vi "Dashboard Main.vi"() -> ()   [LabVIEW 2019]
uses:
  <vilib>/Utility/miscctls.llb/LVRowAndColumnTypeDef.ctl
  <vilib>/event_ctls.llb/eventvkey.ctl
  <vilib>/Rock Robotics/Network Tables/NT Read Numeric Array.vi
  <vilib>/Rock Robotics/WPI/Dashboard/WPI_DashboardLogging Global.vi
panel:
  in  "On/Off  2":bool caption="Solenoid"
  in  "On/Off  2":bool caption="Solenoid"
  in  "On/Off  2":bool caption="Solenoid"
  in  "On/Off  2":bool caption="Solenoid"
  in  "Camera Settings Right":T1={"Frame Rate"=30, "Compression"=30, "Size"=1, "DB Camera Config"=FALSE} {"Frame Rate" scale=1.0..30.0; "Compression" scale=100.0..-1.0; "Size" items=["640x480", "320x240", "160x120"]}
  in  "Camera Name Right":string(combo)="No Camera Selection"
  out "Camera Perf":string
  in  "Camera Settings":T1={"Frame Rate"=30, "Compression"=30, "Size"=1, "DB Camera Config"=FALSE} {"Frame Rate" scale=1.0..30.0; "Compression" scale=100.0..-1.0; "Size" items=["640x480", "320x240", "160x120"]}
  in  "TCP":refnum<k5>
  in  "Rec Mode":enum32{"Stop", "Record", "Playback"}(radio)
  out "Robot IP":string
  out "Image Message":string="Timeout in Camera Communications"
  in  "Dashboard Tab":T2(tab)
  in  "Select Auto":string(combo)="Select Autonomous ..."
  out "NT Connection":bool
  out "MotorChart R":cluster{"Numeric":dbl, "Numeric":dbl}(graph)
  out "MotorChart L":cluster{"Numeric":dbl, "Numeric":dbl}(graph)
  out "MotorSliders R":cluster{"MotorSlide1":dbl, "MotorSlide2":dbl} {"MotorSlide2" scale=-1.0..1.0 scale format="%#_2e"; "MotorSlide1" scale=-1.0..1.0 scale format="%#_2e"}
  out "MotorSliders L":cluster{"MotorSlide1":dbl, "MotorSlide2":dbl} {"MotorSlide2" scale=-1.0..1.0 scale format="%#_2e"; "MotorSlide1" scale=-1.0..1.0 scale format="%#_2e"}
  out "Gyro":dbl(knob) scale=0.0..360.0
  out "JS1 Z":dbl(slide) scale=-1.0..1.0 scale format="%#_2e"
  out "JS1 Graph":cluster{"X":dbl, "Y":dbl}[](graph)
  out "JS1 Buttons":T3
  out "JS2 Z":dbl(slide) scale=-1.0..1.0 scale format="%#_2e"
  out "JS2 Graph":cluster{"X":dbl, "Y":dbl}[](graph)
  out "JS2 Buttons":T3
  out "Mode":T4(ring)=enum."Auto Disabled"
  out "Right Camera Perf":cluster{"Bandwidth (Mbps)":dbl, "FPS":dbl}
  out "Camera Image Right":T5(plugin-control)
  in  "DB/String 9":string
  in  "DB/String 8":string
  in  "DB/String 7":string
  in  "DB/String 6":string
  in  "DB/String 5":string
  in  "DB/String 4":string
  in  "DB/String 3":string
  in  "DB/String 2":string
  in  "DB/String 1":string
  in  "DB/String 0":string
  in  "DB/Slider 0":dbl(slide) scale=0.0..5.0
  in  "DB/Slider 1":dbl(slide) scale=0.0..5.0
  in  "DB/Slider 2":dbl(slide) scale=0.0..5.0
  in  "DB/Slider 3":dbl(slide) scale=0.0..5.0
  out "DB/LED 3":bool
  out "DB/LED 2":bool
  out "DB/LED 1":bool
  out "DB/LED 0":bool
  in  "DB/Button 3":bool
  in  "DB/Button 2":bool
  in  "DB/Button 1":bool
  in  "DB/Button 0":bool caption="New Name"
  in  "Auto Elevator":bool
  out "Current Color":string
  out "Current Trim":dbl
  in  "Trim Start":dbl
  out "Shooter Trim":string
  out "In Camera":bool
  out "No Current Draw":string
  out "Over 250 Amps":bool
  out "Aligned":bool
  out "Wheel at Speed":bool
  out "Ready to Fire":bool
  in  "Auton Delay":dbl
  in  "Autonomous":string(combo)
  out "Elevator Sensor":dbl
  in  "p input":dbl
  out "Left Drive Encoder":string
  out "Shooter Encoder":string
  out "Gyro":string
  out "Limelight-Distance":string
  out "Limelight-TS":string
  out "Limelight-TY":string
  out "Limelight-TX":string
  out "Control Panel Color Sensor":string
  out "Control Panel Encoder":string
  out "Right Drive Encoder":string
  out "Conveyor Motor":string
  out "Right Climber":string
  out "Left Climber":string
  out "Buddy Climb Motor":string
  out "Intake Motor":string
  out "Shooter Motor 2":string
  out "Shooter Motor 1":string
  out "Control Panel":string
  out "Right Drive Motor 2":string
  out "Right Drive Motor 1":string
  out "Left Drive Motor 2":string
  out "Left Drive Motor 1":string
  in  "Test Slider":dbl(slide) scale=0.0..100.0 scale format="%#_3g"
  in  "On/Off":bool caption="Solenoid"
  in  "Test Name":u16(ring) items=["Select the test to run..."]
  in  "Test Tree":string(tree)
  in  "Motor":cluster{"Value":dbl, "Enable":bool} {"Value" scale=-1.0..1.0 scale format="%#_3g"}
  out "Progress":T6 {"Test Progress" scale=0.0..100.0}
  in  "Rev/Fwd":cluster{"Forward":bool, "Reverse":bool}
  in  "Test Ring":u16(ring) items=["Monochrome", "Color"]
  out "Cmd Status":string
  in  "Execute Command":bool
  in  "Command Params":string[][](table)
  in  "Command Selection":i32(listbox)
  in  "CheckList":i32(listbox)
  out "Tree":string(tree)
  out "Camera Image":T5(plugin-control)
  in  "Camera Name":string(combo)="No Camera Selection"
  # "HW"
  # "HW"
  # "Joysticks"
  # "Drive Motors"
  # "Front"
  # "Right"
  # "Left"
  # "Back"
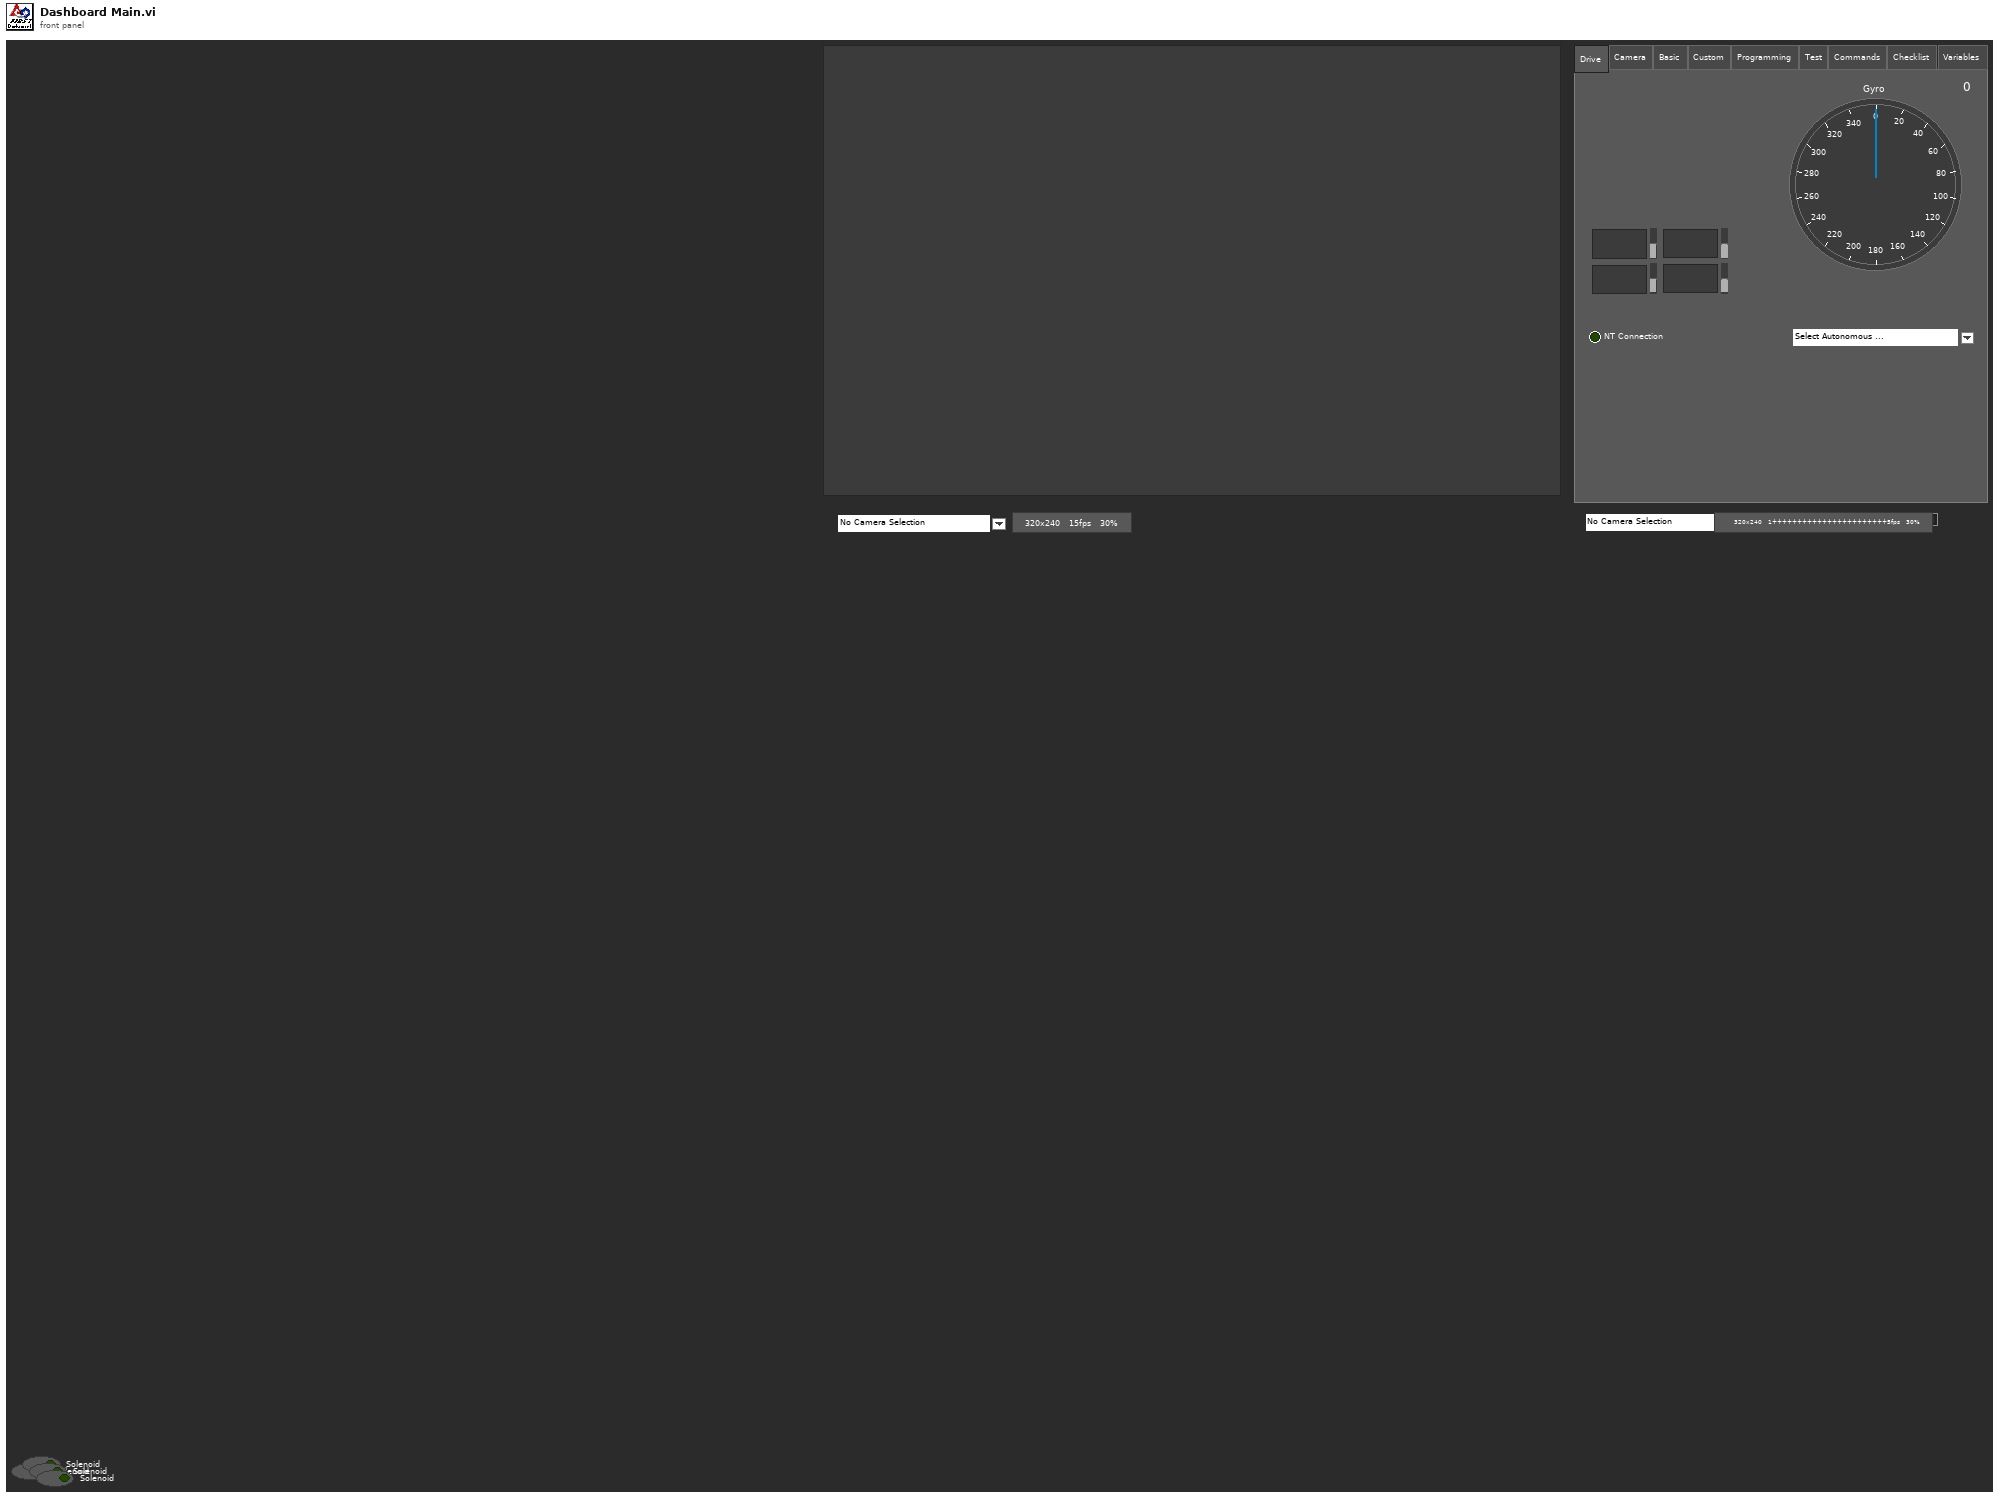
[diagram p1: front panel]
types:
  T1 = cluster{"Frame Rate":i32, "Compression":i32, "Size":u16, "DB Camera Config":bool}
  T2 = enum32{"Drive", "Camera", "Basic", "Custom", "Programming", "Test", "Commands", "Checklist", "Variables"}
  T3 = cluster{bool, bool, bool, bool, bool, bool, bool, bool, bool, bool, bool, bool}
  T4 = enum8{"Tele-Op Disabled", "Tele-Op Enabled", "Auto Disabled", "Auto Enabled", "Test Disabled", "Test Enabled", "Disconnected", "No Code", "E-Stop"}
  T5 = typedef "IMAQ Image.ctl" = refnum<image>
  T6 = cluster{"Test Progress":u8, "Test Progress Text":string}
  T7 = enum32{"Drive", "Camera", "Basic", "Programming", "Custom", "Test", "Commands", "Checklist", "Variables"}
  T8 = cluster{"Save Path":path, "Interval (s)":dbl, "Keep":i32}
  T9 = typedef "Image Type" = u32
  T10 = cluster{"IDs":cluster{"RPC field ID":u16, "Unique ID":u16}, "String":string}
  T11 = cluster{"Error Strings":string, "Disable Counts":cluster{u16, u16}, "Rail Faults":cluster{u16, u16, u16}, "Robot IP":string, "DB Mode":u8, "Event Info":cluster{"Name":string, "Type":u8, "Number":u16, "Replay":u8}}
  T12 = cluster{"Storage":cluster{"Disk Free":u64, "RAM Block":u32, "RAM free":u32}, "CPU Utilization":cluster{"CPU % ISR":sgl, "CPU % Time Crit":sgl, "CPU % Timed Str":sgl, "CPU % High":sgl, "CPU % Above":sgl, "CPU % Normal":sgl, "CPU % Low":sgl}, "CAN":cluster{"% Bus Utilization":sgl, "Bus Off Cnt":u32, "TX_FIFO Full Cnt":u32, "Receive Error Cnt":u8, "Transmit Error Cnt":u8}, "HID":cluster{"HID Outputs":u32, "Rumble Low":u16, "Rumble High":u16}[]}
  T13 = cluster{"Status bits":cluster{"Test Mode":bool, "Autonomous":bool, "Enabled":bool, "Code Start":bool, "Brownout":bool, "Reserved 2":bool, "Reserved 3":bool, "E-Stop":bool}, "Code Trace":cluster{"Disabled":bool, "TeleOp":bool, "Auto":bool, "Test":bool}, "Controller Type":enum16{"unknown", "cRIO", "roboRio"}, "Code?":enum16{"unknown", "noCode", "code"}, "Battery V":dbl}
  T14 = cluster{"Control Bits":cluster{"TestMode":bool, "Autonomous":bool, "Enabled":bool, "FMS Present":bool, bool, bool, bool, "E-Stop":bool}, "Team Station ":u8, "Countdown":sgl, "Joystick Values":cluster{"Axes":dbl[], "Buttons":bool[], "POVs":i16[]}[]}
  T15 = cluster{"Axes":dbl[], "Buttons":bool[], "POVs":i16[]}[]
  T16 = cluster{"Axes":dbl[], "Buttons":bool[], "POVs":i16[]}
  T17 = cluster{"Buttons[0]":bool, "Buttons[1]":bool, "Buttons[2]":bool, "Buttons[3]":bool, "Buttons[4]":bool, "Buttons[5]":bool, "Buttons[6]":bool, "Buttons[7]":bool, "Buttons[8]":bool, "Buttons[9]":bool, "Buttons[10]":bool, "Buttons[11]":bool}
  T18 = cluster{"Camera Image":refnum<vi>, "Dashboard Tab":refnum<vi>, "Background":refnum<vi>, "Rec Mode":refnum<vi>, "Test Slider":refnum<vi>, "On/Off ":refnum<vi>, "Test Ring":refnum<vi>, "Rev/Fwd":refnum<vi>, "Test Name":refnum<vi>, "Motor":refnum<vi>, "Progress":refnum<vi>, "CheckList":refnum<vi>, "Tree":refnum<vi>, "Test Tree":refnum<vi>, "Command Params":refnum<vi>, "Command Selection":refnum<vi>, "Execute Command":refnum<vi>, "Cmd Status":refnum<vi>, "Camera Settings":refnum<vi>, "Camera Name":refnum<vi>, "Camera Perf":refnum<vi>, "Camera Settings Right":refnum<vi>, "Camera Name Right":refnum<vi>, "Camera Image Right":refnum<vi>}
  T19 = cluster{"Global Rectangle":i32[], "Contours":cluster{"Contour Type":u32, "ROI Type":u32, "Points":i32[]}[]}
  T20 = cluster{"Camera Name":string, string, "Saved DB Images Info":cluster{"Save Path":path, "Interval (s)":dbl, "Keep":i32}}
  T21 = cluster{"Camera Name Right":string, string, "Saved DB Images Info":cluster{"Save Path":path, "Interval (s)":dbl, "Keep":i32}}
  T22 = cluster{"Operation":enum16{"Update", "Clear"}, "Color Box":u32}[]
  T23 = typedef "eventvkey.ctl" = enum16{"ASCII", "Enter", "Return", "Shift", "Ctrl", "Alt", "Cmd", "Opt", "Caps", "NumLock", "Clear", "Break", "Up", "Down", "Left", "Right", "Insert", "Delete", "Home", "End", "PageUp", "PageDown", "Escape", "Help", "Pause", "ScrollLock", "F1", "F2", "F3", "F4", "F5", "F6", "F7", "F8", "F9", "F10", "F11", "F12", "F13", "F14", "F15", "F16", "F17", "F18", "F19", "F20", "F21", "F22", "F23", "F24", "Play", "VolumeUp", "VolumeDown", "Mute", "Two Byte Char"}
  T24 = cluster{"Image Size":bool, "Image Type":bool, "Pixel Value":bool, "ROI Information":bool, "Zoom Factor":bool}
  T25 = cluster{"Operation":enum16{"Update", "Clear"}, "Color Box":u32}
  T26 = typedef "LVRowAndColumnTypeDef.ctl" = cluster{"Row":i32, "Column":i32}
  T27 = cluster{"Shift":bool, "Ctrl":bool, "Alt":bool, "Cmd":bool, "Opt":bool}
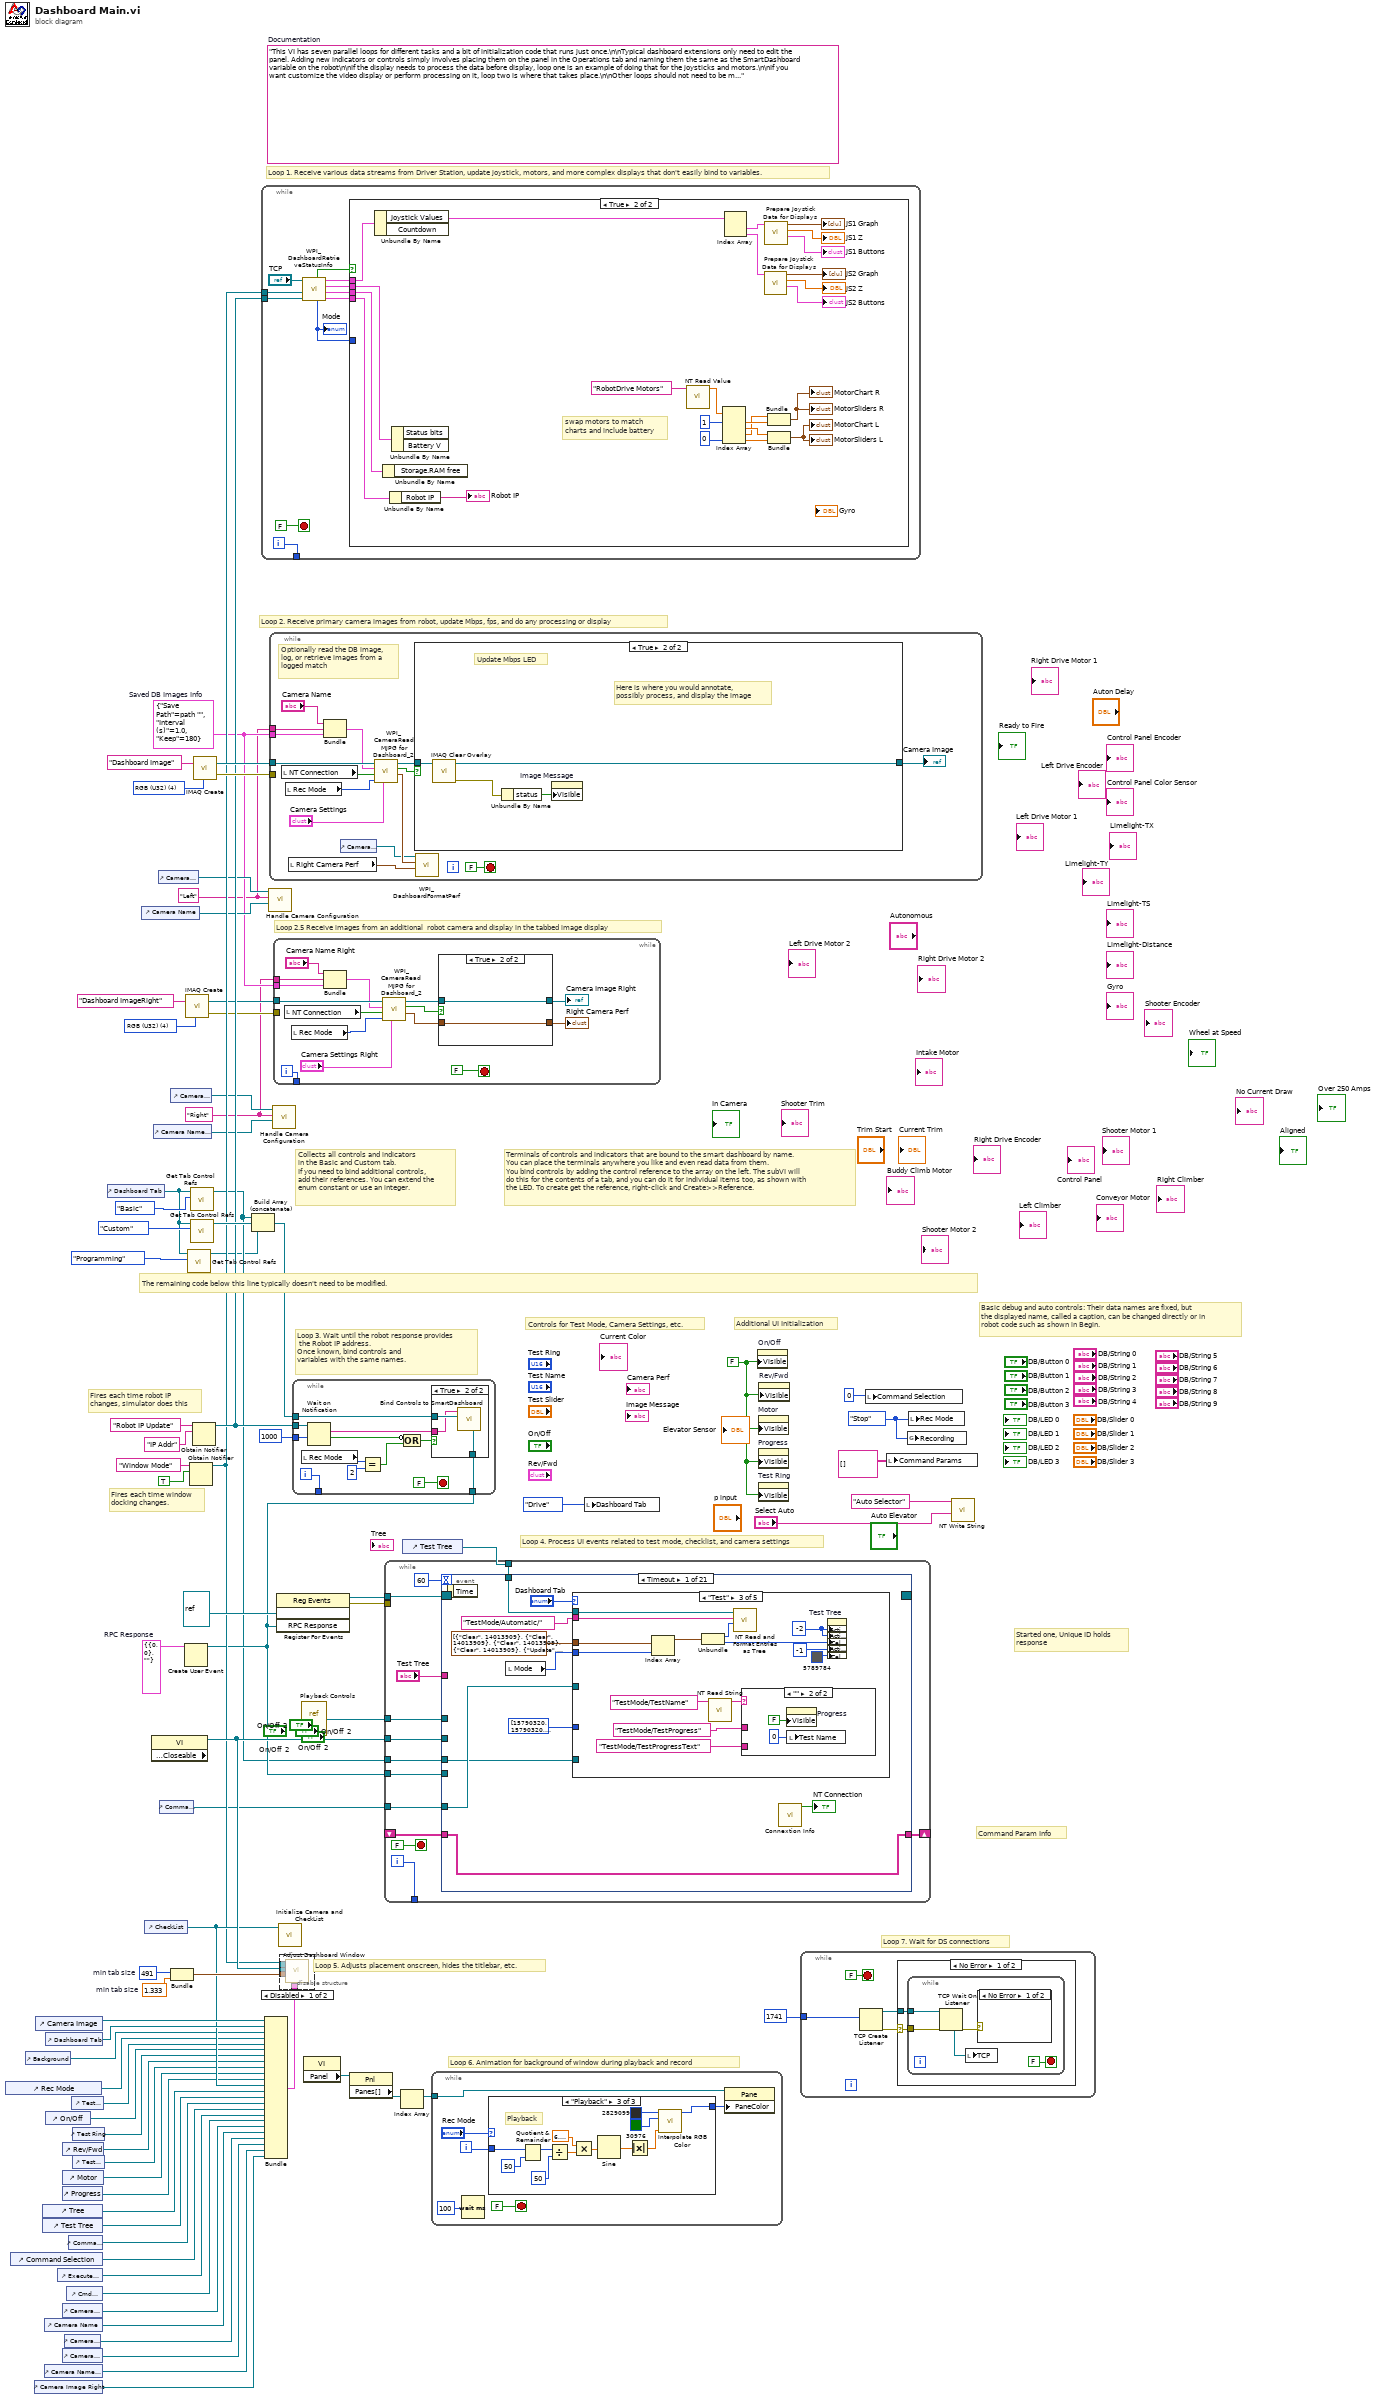
[diagram p0: block diagram]
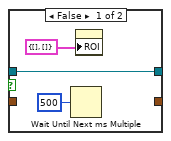
[diagram p3: hidden frame]
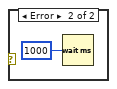
[diagram p4: hidden frame]
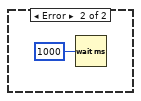
[diagram p5: hidden frame]
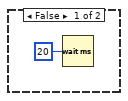
[diagram p6: hidden frame]
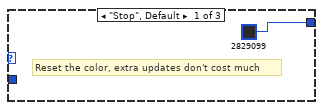
[diagram p7: hidden frame]
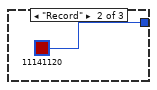
[diagram p8: hidden frame]
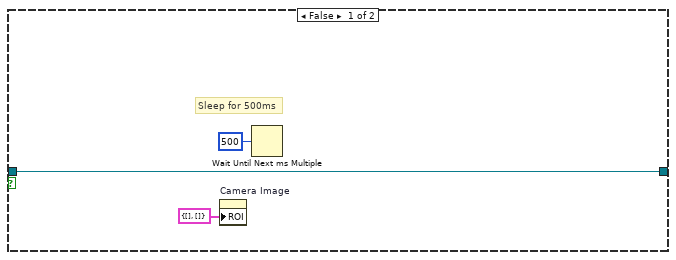
[diagram p10: hidden frame]
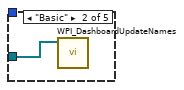
[diagram p12: hidden frame]
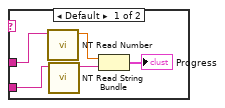
[diagram p13: hidden frame]
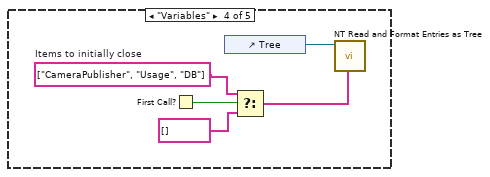
[diagram p14: hidden frame]
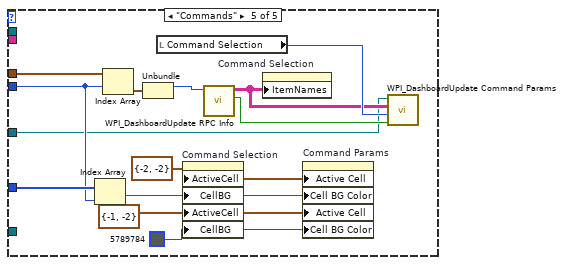
[diagram p15: hidden frame]
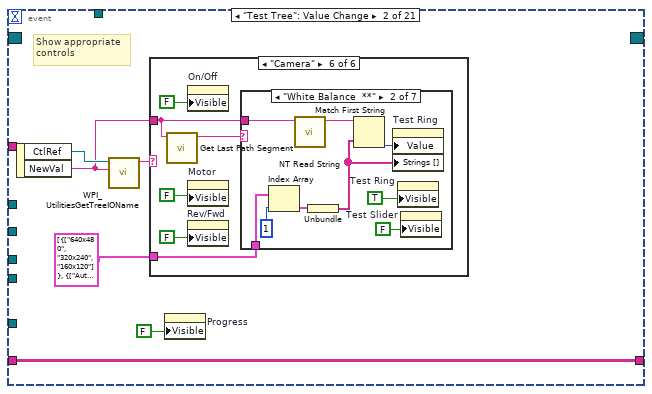
[diagram p16: hidden frame]
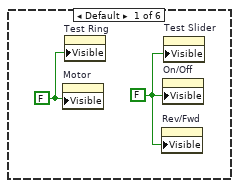
[diagram p17: hidden frame]
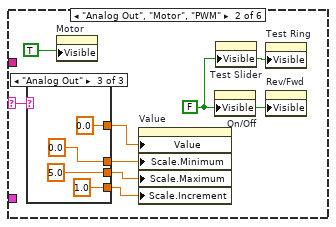
[diagram p18: hidden frame]
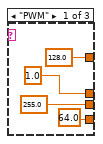
[diagram p19: hidden frame]
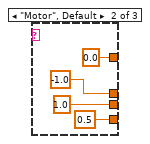
[diagram p20: hidden frame]
diagram:
  w7 = T8 {"Save Path"=path "", "Interval (s)"=1.0, "Keep"=180}  # Saved DB Images Info
  w6 = "Right"
  w5 = "Left"
  w17 = T9 4 items=["Grayscale (U8)", "Grayscale (I16)", "Grayscale (SGL)", "Complex (CSG)", "RGB (U32)", "HSL (U32)", "RGB (U64)"] ("Image Type")
  w33 = T10 {"IDs"={"RPC field ID"=0, "Unique ID"=0}, "String"=""}  # RPC Response
  w55 = 491  # min tab size
  w54 = 1.333  # min tab size
  w61 = enum32{"Stop", "Record", "Playback"}."Stop" ("Rec Mode")
  w40 = FALSE ("Visible")
  (unwired) "This VI has seven parallel loops for different tasks and a bit of initialization code that runs just once.\n\nTypical dashboard extensions only need to edit the panel. Adding new indicators or controls simply involves placing them on the panel in the Operations tab and naming them the same as the SmartDashboard variable on the robot\n\nIf the display needs to process the data before display, loop one is an example of doing that for the joysticks and motors.\n\nIf you want customize the video display or perform processing on it, loop two is where that takes place.\n\nOther loops should not need to be modified. They are pretty standard, and document the task they perform."  # Documentation
  w78 = T9 4 items=["Grayscale (U8)", "Grayscale (I16)", "Grayscale (SGL)", "Complex (CSG)", "RGB (U32)", "HSL (U32)", "RGB (U64)"] ("Image Type")
  # "Loop 2.5 Receive images from an additional  robot camera and display in the tabbed image display"
  # "Command Param Info"
  # "Started one, Unique ID holds\nresponse"
  # "Loop 7. Wait for DS connections"
  # "Basic debug and auto controls: Their data names are fixed, but\nthe displayed name, called a caption, can be changed directly or in\nrobot code such as shown in Begin."
  # "Controls for Test Mode, Camera Settings, etc."
  # "Additional UI Initialization"
  # "Loop 6. Animation for background of window during playback and record"
  # "Fires each time robot IP\nchanges, simulator does this"
  # "Fires each time window\ndocking changes."
  # "Collects all controls and indicators\nin the Basic and Custom tab.\nIf you need to bind additional controls,\nadd their references. You can extend the\nenum constant or use an integer."
  # "The remaining code below this line typically doesn't need to be modified."
  # "Loop 4. Process UI events related to test mode, checklist, and camera settings"
  # "Terminals of controls and indicators that are bound to the smart dashboard by name.\nYou can place the terminals anywhere you like and even read data from them.\nYou bind controls by adding the control reference to the array on the left. The subVI will\ndo this for the contents of a tab, and you can do it for individual items too, as shown with\nthe LED. To create get the reference, right-click and Create>>Reference."
  # "Loop 3. Wait until the robot response provides\n the Robot IP address.\nOnce known, bind controls and\nvariables with the same names."
  # "Loop 5. Adjusts placement onscreen, hides the titlebar, etc."
  # "Loop 1. Receive various data streams from Driver Station, update joystick, motors, and more complex displays that don't easily bind to variables."
  # "Loop 2. Receive primary camera images from robot, update Mbps, fps, and do any processing or display"
  n1 = control-ref of="Rec Mode"() -> (w46:refnum<vi>)
  n2 = control-ref of="Command Selection"() -> (w32:refnum<vi>)
  n3 = control-ref of="Background"() -> (w4:refnum<vi>)
  n4 = control-ref of="Camera Image Right"() -> (w10:refnum<vi>)
  n5 = control-ref of="Camera Image"() -> (w57:refnum<vi>)
  n6 = control-ref of="Tree"() -> (w50:refnum<vi>)
  n7 = control-ref of="Test Tree"() -> (w49:refnum<vi>)
  n8 = control-ref of="Camera Name"() -> (w23:refnum<vi>)
  n9 = control-ref of="Camera Name Right"() -> (w11:refnum<vi>)
  n10 = control-ref of="On/Off"() -> (w44:refnum<vi>)
  n11 = control-ref of="Dashboard Tab"() -> (w56:refnum<vi>)
  n12 = control-ref of="Execute Command"() -> (w34:refnum<vi>)
  n13 = control-ref of="Progress"() -> (w41:refnum<vi>)
  n14 = control-ref of="Camera Settings"() -> (w24:refnum<vi>)
  n15 = control-ref of="Camera Settings Right"() -> (w12:refnum<vi>)
  n16 = control-ref of="Rev/Fwd"() -> (w42:refnum<vi>)
  n17 = control-ref of="Motor"() -> (w47:refnum<vi>)
  n18 = control-ref of="Camera Perf"() -> (w22:refnum<vi>)
  n19 = control-ref of="Cmd Status"() -> (w28:refnum<vi>)
  n20 = control-ref of="Command Params"() -> (w35:refnum<vi>)
  n21 = control-ref of="Test Slider"() -> (w45:refnum<vi>)
  n22 = control-ref of="Test Ring"() -> (w43:refnum<vi>)
  n23 = control-ref of="Test Name"() -> (w48:refnum<vi>)
  n24 = control-ref of="Dashboard Tab"() -> (w2:refnum<vi>)
  n25 = control-ref of="Camera Name"() -> (w25:refnum<vi>)
  n26 = control-ref of="CheckList"() -> (w51:refnum<vi>)
  n27 = property class="VI" props=["Front Panel.Closeable"]() -> (reference out=w60:refnum<vi>)  [unwired: 2 in, 2 out]
  n28 = control-ref of="Camera Name Right"() -> (w13:refnum<vi>)
  n29 = control-ref of="Camera Settings"() -> (w26:refnum<vi>)
  n30 = control-ref of="Command Params"() -> (w27:refnum<vi>)
  n31 = control-ref of="Camera Settings Right"() -> (w14:refnum<vi>)
  n32 = Bundle("min tab size"=w55, "min tab size"=w54) -> (w53:cluster{"min tab size":i32, "min tab size":dbl})  [unwired: 1 in]
  n33 = Create User Event(user event datatype=w33) -> (user event=w29:refnum<user-event>)  [unwired: 1 in, 1 out]
  n34 = call "IMAQ Create"("Image Name"="Dashboard ImageRight", "Image Type"=w17) -> ("New Image"=w16:T5, "error out"=w15:errorcluster)  [unwired: 2 in, 1 out]
  n35 = call <vilib>:"Get Tab Control Refs.vi"("Page Index"=T7."Programming" ("Dashboard Tab"), "TabControl in"=w2) -> ("ControlsOnPage"=w1:refnum<vi>[])  [unwired: 9 in]
  n36 = Obtain Notifier(name (unnamed)="Window Mode", notification data type=TRUE) -> (notifier out=w38:refnum<notifier>)  [unwired: 2 in, 2 out]
  n37 = call <vilib>:"Get Tab Control Refs.vi"("Page Index"=T7."Basic" ("Dashboard Tab"), "TabControl in"=w2) -> ("ControlsOnPage"=w21:refnum<vi>[])  [unwired: 9 in]
  n38 = call <vilib>:"Get Tab Control Refs.vi"("Page Index"=T7."Custom" ("Dashboard Tab"), "TabControl in"=w2) -> ("ControlsOnPage"=w59:refnum<vi>[])  [unwired: 9 in]
  n39 = Obtain Notifier(name (unnamed)="Robot IP Update", notification data type="IP Addr" ("name (unnamed)")) -> (notifier out=w39:refnum<notifier>)  [unwired: 2 in, 2 out]
  n40 = call "IMAQ Create"("Image Name"="Dashboard Image", "Image Type"=w78) -> ("New Image"=w76:T5, "error out"=w75:errorcluster)  [unwired: 2 in, 1 out]
  n41 = Build Array (concatenate)(w21, w59, w1) -> (w58:refnum<vi>[])
  n42 = while {
    tunnel: [w88] -> _
    tunnel: w39 -> [w82]
    tunnel: w38 -> [w79]
    i -> [w88]
    stop <- FALSE stop-if-true
    n43 = call <vilib>:"WPI_DashboardRetrieveStatusInfo.vi"("Binding Refnum"=w82, "Window Mode Notifier"=w79, "TCP Cnx"="TCP") -> ("Power and Errors"=w83:T11, "Robot Metrics"=w86:T12, "Status Info"=w87:T13, "Control Info"=w84:T14, "Robot Mode"=w81:T4, "Process?"=w85:bool)  [unwired: 3 in]
    "Mode" <- w81
    n44 = case shown="True" w85 {
      tunnel: w87 -> [_ w114]
      tunnel: w86 -> [_ w113]
      tunnel: w84 -> [_ w112]
      tunnel: w83 -> [_ w111]
      tunnel: w81 -> [_ _]
      frame False {
        n45 = Wait (ms)(milliseconds to wait=u32 20) -> ()  [unwired: 1 out]
      }
      frame True {
        # "swap motors to match\ncharts and include battery"
        n46 = Unbundle By Name(w112) -> ("Joystick Values"=w102:T15)  [unwired: 1 out]
        n47 = Unbundle By Name(w113) -> ()  [unwired: 1 out]
        n48 = Unbundle By Name(w111) -> ("Robot IP"=→"Robot IP":string)
        n49 = Unbundle By Name(w114) -> ()  [unwired: 2 out]
        n50 = call-poly <vilib>:"NT Read Value.vi"("Name"="RobotDrive Motors") -> ("Numeric Array"=w92:dbl[])  [unwired: 9 in, 1 out]
        n51 = Index Array(array=w92, index #1=1, index #4=0) -> (element #1=w106:dbl, element #2=w107:dbl, element #3=w105:dbl, element #4=w110:dbl)  [unwired: 2 in]
        n52 = Index Array(array=w102) -> (element #1=w101:T16, element #2=w97:T16)  [unwired: 2 in]
        n53 = call "Prepare Joystick Data for Displays.vi"("Joystick Values"=w97) -> ("Buttons"=→"JS2 Buttons":T17, "Z Axis"=→"JS2 Z":dbl, "Cartesian Data"=→"JS2 Graph":cluster{"X axis":dbl, "X axis":dbl}[])  [unwired: 8 in]
        n54 = call "Prepare Joystick Data for Displays.vi"("Joystick Values"=w101) -> ("Buttons"=→"JS1 Buttons":T17, "Z Axis"=→"JS1 Z":dbl, "Cartesian Data"=→"JS1 Graph":cluster{"X axis":dbl, "X axis":dbl}[])  [unwired: 8 in]
        n55 = Bundle("Numeric"=w105, "Numeric"=w106) -> (→"MotorChart R" →"MotorSliders R":cluster{"Numeric":dbl, "Numeric":dbl})  [unwired: 1 in]
        n56 = Bundle("Numeric"=w107, "Numeric"=w110) -> (→"MotorChart L" →"MotorSliders L":cluster{"Numeric":dbl, "Numeric":dbl})  [unwired: 1 in]
      }
    }
  }
  n57 = Bundle("Camera Image"=w57, "Dashboard Tab"=w56, "Background"=w4, "Rec Mode"=w46, "Test Slider"=w45, "On/Off"=w44, "Test Ring"=w43, "Rev/Fwd"=w42, "Test Name"=w48, "Motor"=w47, "Progress"=w41, "CheckList"=w51, "Tree"=w50, "Test Tree"=w49, "Command Params"=w35, "Command Selection"=w32, "Execute Command"=w34, "Cmd Status"=w28, "Camera Settings"=w24, "Camera Name"=w23, "Camera Perf"=w22, "Camera Settings Right"=w12, "Camera Name Right"=w11, "Camera Image Right"=w10) -> (w52:T18)  [unwired: 1 in]
  n58 = call "Handle Camera Configuration.vi"("CameraNameRef"=w25, "Display Name"=w5, "ClusterRef"=w26) -> ()  [unwired: 9 in]
  n59 = while {
    tunnel: w76 -> [w128]
    tunnel: w75 -> [_]
    tunnel: w7 -> [w121]
    tunnel: w5 -> [w118]
    stop <- FALSE stop-if-true
    # "Optionally read the DB image,\nlog, or retrieve images from a\nlogged match"
    n60 = local read "NT Connection"() -> (w122:bool)
    n61 = local read "Rec Mode"() -> (w125:enum32{"Stop", "Record", "Playback"})
    n62 = local read "Right Camera Perf"() -> (w116:cluster{"Bandwidth (Mbps)":dbl, "FPS":dbl})
    n63 = Bundle("Camera Name"="Camera Name", w118, "Saved DB Images Info"=w121) -> (w120:T20)  [unwired: 1 in]
    n64 = control-ref of="Camera Perf"() -> (w115:refnum<vi>)
    n65 = call <vilib>:"WPI_CameraRead MJPG for Dashboard_2.vi"("Camera Settings"="Camera Settings", "Rec Mode"=w125, "NT Connection"=w122, "Capture Info"=w120, "Image in"=w128) -> ("perf info"=w117:cluster{"Bandwidth (Mbps)":dbl, "fps":dbl}, "Active"=w126:bool, "Image\\ out"=w127:T5)  [unwired: 4 in]
    n66 = case shown="True" w126 {
      tunnel: w127 -> [w131 w134]
      tunnel: [w131 w133] -> w123
      frame False {
        # "Sleep for 500ms"
        n67 = property on="Camera Image" class="ImageControl"("ROI"=T19 {"Global Rectangle"=[], "Contours"=[]}) -> ()  [unwired: 2 in, 2 out]
        n68 = Wait Until Next ms Multiple(millisecond multiple=u32 500) -> ()  [unwired: 1 out]
      }
      frame True {
        # "Here is where you would annotate,\npossibly process, and display the image"
        # "Update Mbps LED"
        n69 = call "IMAQ Clear Overlay"("Image"=w134) -> ("error out"=w135:errorcluster, "Image Out"=w133:T5)  [unwired: 2 in, 7 out]
        n70 = Unbundle By Name(w135) -> ("status"=w136:bool)
        n71 = property on="Image Message" class="Str"("Visible"=w136) -> ()  [unwired: 2 in, 2 out]
      }
    }
    "Camera Image" <- w123
    n72 = call <vilib>:"WPI_DashboardFormatPerf.vi"("Right Camera Perf"=w116, "Performance"=w117, "String in"=w115) -> ()  [unwired: 9 in]
  }
  n73 = call "Handle Camera Configuration.vi"("CameraNameRef"=w13, "Display Name"=w6, "ClusterRef"=w14) -> ()  [unwired: 9 in]
  n74 = while {
    tunnel: w16 -> [w151]
    tunnel: w15 -> [_]
    tunnel: [w146] -> _
    tunnel: w7 -> [w142]
    tunnel: w6 -> [w139]
    i -> [w146]
    stop <- FALSE stop-if-true
    n75 = local read "NT Connection"() -> (w143:bool)
    n76 = local read "Rec Mode"() -> (w150:enum32{"Stop", "Record", "Playback"})
    n77 = Bundle("Camera Name Right"="Camera Name Right", w139, "Saved DB Images Info"=w142) -> (w141:T21)  [unwired: 1 in]
    n78 = call <vilib>:"WPI_CameraRead MJPG for Dashboard_2.vi"("Camera Settings"="Camera Settings Right", "Rec Mode"=w150, "NT Connection"=w143, "Capture Info"=w141, "Image in"=w151) -> ("perf info"=w137:cluster{"Bandwidth (Mbps)":dbl, "fps":dbl}, "Active"=w145:bool, "Image\\ out"=w148:T5)  [unwired: 4 in]
    n79 = case shown="True" w145 {
      tunnel: w148 -> [w153 w156]
      tunnel: [w153 w156] -> w144
      tunnel: [_ w155] -> w138
      tunnel: w137 -> [_ w155]
      frame False {
        n80 = Wait Until Next ms Multiple(millisecond multiple=u32 500) -> ()  [unwired: 1 out]
        n81 = property on="Camera Image Right" class="ImageControl"("ROI"=T19 {"Global Rectangle"=[], "Contours"=[]}) -> ()  [unwired: 2 in, 2 out]
      }
      frame True {
      }
    }
    "Camera Image Right" <- w144
    "Right Camera Perf" <- w138
  }
  n82 = register-events(refnum<vi> refnum, w29) -> (reference out=w65:refnum<event-registration>, error out=w64:errorcluster)  [unwired: 2 in]
  n83 = call "Initialize Camera and CheckList.vi"("ListBox in"=w51) -> ()  [unwired: 11 in]
  n84 = disable-structure shown="Disabled" {
    disable-tunnel: w60 -> [w160 _]
    disable-tunnel: w53 -> [w159 _]
    disable-tunnel: w52 -> [w158 _]
    disable-tunnel: w38 -> [w157 _]
    frame Disabled {
      n85 = call "Adjust Dashboard Window.vi"("Sizing Refnums"=w158, "Size Constraints"=w159, "VI"=w160, "WIn Mode"=w157) -> ()  [unwired: 8 in]
    }
    frame Enabled {
    }
  }
  n86 = while {
    tunnel: w58 -> [w172]
    tunnel: w39 -> [w170]
    tunnel: [w168] -> _
    tunnel: u32 1000 ("milliseconds to wait") -> [w167]
    tunnel: w29 -> [w161]
    i -> [w168]
    stop <- FALSE stop-if-true
    n87 = local read "Rec Mode"() -> (w163:enum32{"Stop", "Record", "Playback"})
    n88 = Wait on Notification(notifier=w170, timeout in ms (-1)=w167) -> (notification=w169:string, timed out?=w165:bool)  [unwired: 2 in, 2 out]
    n89 = Equal?(x=w163, y=u16 2 ("Rec Mode")) -> (x = y?=w164:bool)
    n90 = Compound Arithmetic op=OR(invert w165, w164) -> (w166:bool)
    n91 = case shown="True" w166 {
      tunnel: w172 -> [_ w175]
      tunnel: w169 -> [_ w174]
      tunnel: w161 -> [_ w173]
      frame False {
      }
      frame True {
        n92 = call <vilib>:"Bind Controls to SmartDashboard.vi"("RPC ref"=w173, "Bound Control Refs"=w175, "Server IP Address"=w174) -> ()  [unwired: 9 in]
      }
    }
  }
  n93 = vi-ref "Playback Controls.vi"() -> (w66:refnum<vi>)
  n94 = property class="VI"() -> ("Panel"=w68:refnum<vi>)  [unwired: 2 in, 2 out]
  n95 = property class="Pnl"(reference=w68) -> ("Panes[]"=w69:refnum<vi>[])  [unwired: 1 in, 2 out]
  n96 = Index Array(array=w69) -> (element=w67:refnum<vi>)  [unwired: 1 in]
  n97 = control-ref of="Test Tree"() -> (w70:refnum<vi>)
  n98 = while {
    tunnel: [w185] -> _
    tunnel: w70 -> [w184]
    tunnel: w66 -> [w183]
    tunnel: w65 -> [w182]
    tunnel: w64 -> [_]
    tunnel: w60 -> [w181]
    tunnel: w29 -> [w180]
    tunnel: w27 -> [w179]
    shift-right: [w178] -> _
    shift-left: _ -> [w177]
    tunnel: w21 -> [w176]
    i -> [w185]
    stop <- FALSE stop-if-true
    n99 = event shown="[0] Timeout" {
      selector: w182 -> [_ _ _ _ _ _ _ _ _ _ _ _ _ _ _ _ _ _ _ _ _]
      dyn-events: [_ _ _ _ _ _ _ _ _ _ _ _ _ _ _ _ w445 _ _ _ _] -> _
      timeout: u32 60 ("milliseconds to wait") -> [_ _ _ _ _ _ _ _ _ _ _ _ _ _ _ _ _ _ _ _ _]
      tunnel: w184 -> [w197 _ _ _ _ _ _ _ _ _ _ _ _ _ _ _ _ _ _ _ _]
      tunnel: "Test Tree" -> [_ _ _ _ _ _ _ _ _ _ _ w412 w420 w422 w426 w434 _ _ _ _ _]
      tunnel: w183 -> [_ _ _ _ _ _ _ _ _ _ _ _ _ _ _ _ w447 _ w465 _ _]
      tunnel: w181 -> [_ _ _ _ _ _ _ _ _ _ _ _ _ _ _ _ w443 _ _ _ _]
      tunnel: w180 -> [_ _ _ _ _ _ _ _ _ _ _ _ _ _ _ _ w441 _ _ _ _]
      tunnel: w179 -> [w192 _ _ _ _ _ w363 _ _ _ _ _ _ _ _ _ _ _ _ _ _]
      tunnel: [w191 w240 w342 w347 w356 w360 w361 w370 w380 w387 w399 w411 w418 w421 w425 w433 w440 w460 w462 w466 w479] -> w178
      tunnel: w177 -> [w191 w240 w342 w347 w356 w360 w361 _ _ w387 w399 w411 w418 w421 w425 w433 w440 w460 w462 w466 w479]
      tunnel: w176 -> [w189 _ _ _ _ _ _ _ _ _ _ _ _ _ _ _ _ _ _ _ _]
      event Timeout {
        n100 = event-data() -> ()  [unwired: 1 in, 1 out]
        n101 = local read "Mode"() -> (w194:T4)
        n102 = case shown="\"Test\"" "Dashboard Tab" {
          tunnel: w197 -> [_ _ w213 _ _]
          tunnel: "TestMode/Automatic/" ("Name Pattern") -> [_ _ w212 _ _]
          tunnel: T22 [{"Operation"=enum."Clear", "Color Box"=14013909}, {"Operation"=enum."Clear", "Color Box"=14013909}, {"Operation"=enum."Clear", "Color Box"=14013909}, {"Operation"=enum."Clear", "Color Box"=14013909}, {"Operation"=enum."Update", "Color Box"=14013909}, {"Operation"=enum."Update", "Color Box"=16777215}, {"Operation"=enum."Clear", "Color Box"=14013909}, {"Operation"=enum."Clear", "Color Box"=14013909}, {"Operation"=enum."Clear", "Color Box"=14013909}] -> [_ _ w205 _ w233]
          tunnel: w194 -> [_ _ w204 _ w232]
          tunnel: u32[] [15790320, 15790320, 15790320, 15790320, 16777215, 16777215, 15790320, 15790320, 15790320] -> [_ _ _ _ w238]
          tunnel: w192 -> [_ _ _ _ w226]
          tunnel: w189 -> [_ w199 _ _ _]
          frame "Custom", Default {
          }
          frame "Basic" {
            n103 = call <vilib>:"WPI_DashboardUpdateNames.vi"("Controls on Tab"=w199) -> ()  [unwired: 11 in]
          }
          frame "Test" {
            w211 = -2 ("Active Item:Row Number")
            n104 = Index Array(array=w205, index=w204) -> (element=w206:T25)
            n105 = Unbundle(w206) -> ("Operation"=w207:enum16{"Update", "Clear"}, "Color Box"=w208:u32)
            n106 = call <vilib>:"NT Read String.vi"("Name"="TestMode/TestName") -> ("String"=w202:string)  [unwired: 9 in, 1 out]
            n107 = call <vilib>:"NT Read and Format Entries as Tree.vi"("Operation"=w207, "Name Pattern"=w212, "Tree Refnum"=w213) -> ()  [unwired: 7 in, 2 out]
            n108 = case shown="\"\"" w202 {
              tunnel: "TestMode/TestProgress" ("Name") -> [w215 _]
              tunnel: "TestMode/TestProgressText" ("Name") -> [w214 _]
              frame Default {
                n109 = call <vilib>:"NT Read Number.vi"("Name"=w215) -> ("Numeric"=w216:dbl)  [unwired: 9 in, 1 out]
                n110 = call <vilib>:"NT Read String.vi"("Name"=w214) -> ("String"=w217:string)  [unwired: 9 in, 1 out]
                n111 = Bundle("Numeric"=w216, "String"=w217) -> (→"Progress":cluster{"Numeric":dbl, "String":string})  [unwired: 1 in]
              }
              frame "" {
                n112 = property on="Progress" class="Clust (strict)"("Visible"=FALSE) -> ()  [unwired: 2 in, 2 out]
                n113 = local write "Test Name"(u16 0) -> ()
              }
            }
            n114 = property on="Test Tree" class="Tree (strict)"("Active Item Row Number"=w211, "ActiveColNum"=w211, "CellBG"=w208, "Active Item Row Number"=-1 ("Active Item:Row Number"), "CellBG"=u32 5789784 ("Color Box")) -> ()  [unwired: 2 in, 2 out]
          }
          frame "Variables" {
            w223 = string[] ["CameraPublisher", "Usage", "DB"]  # Items to initially close
            n115 = First Call?() -> (First Call?: T/F=w224:bool)
            n116 = control-ref of="Tree"() -> (w225:refnum<vi>)
            n117 = Select(t=w223, s=w224, f=string[] []) -> (s? t:f=w221:string[])
            n118 = call <vilib>:"NT Read and Format Entries as Tree.vi"("Tags to  Close"=w221, "Tree Refnum"=w225) -> ()  [unwired: 8 in, 2 out]
          }
          frame "Commands" {
            w234 = u32 5789784 ("Color Box")
            w235 = T26 {"Row"=-1, "Column"=-2} ("Active Cell:Active Cell")
            w237 = T26 {"Row"=-2, "Column"=-2} ("Active Cell:Active Cell")
            n119 = Index Array(array=w238, index=w232) -> (element=w236:u32)
            n120 = Index Array(array=w233, index=w232) -> (element=w231:T25)
            n121 = Unbundle(w231) -> ("Operation"=w230:enum16{"Update", "Clear"})  [unwired: 1 out]
            n122 = local read "Command Selection"() -> (w229:i32)
            n123 = property on="Command Selection" class="MCListbox (strict)"("ActiveCell"=w237, "CellBG"=w236, "ActiveCell"=w235, "CellBG"=w234) -> ()  [unwired: 2 in, 2 out]
            n124 = call <vilib>:"WPI_DashboardUpdate RPC Info.vi"("Operation"=w230) -> ("update"=w228:bool, "commands"=w227:string[][])  [unwired: 9 in]
            n125 = property on="Command Selection" class="MCListbox (strict)"("ItemNames"=w227) -> ()  [unwired: 2 in, 2 out]
            n126 = property on="Command Params" class="Tbl (strict)"("Active Cell"=w237, "Cell BG Color"=w236, "Active Cell"=w235, "Cell BG Color"=w234) -> ()  [unwired: 2 in, 2 out]
            n127 = call <vilib>:"WPI_DashboardUpdate Command Params.vi"("Update"=w228, "NewVal"=w229, "Commands"=w227, "Param Tbl"=w226) -> ()  [unwired: 7 in, 1 out]
          }
        }
        n128 = call <vilib>:"Connextion Info.vi"() -> ("Connected"=→"NT Connection":bool)  [unwired: 10 in, 1 out]
      }
      event "Test Tree": Value Change {
        # "Show appropriate\ncontrols"
        n129 = event-data() -> ("CtlRef"=w243:refnum<vi>, "NewVal"=w241:string)  [unwired: 1 in]
        n130 = call <vilib>:"WPI_UtilitiesGetTreeIOName.vi"("NewVal"=w241, "TreeControl in"=w243) -> ("I/O Name"=w244:string)  [unwired: 9 in]
        n131 = case shown="\"Camera\"" w244 {
          selector: w244 -> [_ w251 _ w273 w282 _]
          tunnel: w241 -> [_ _ w270 w272 _ w289]
          tunnel: cluster{string[]}[] [{["640x480", "320x240", "160x120"]}, {["Auto", "Fixed indoor", "Fixed outdoor 1", "Fixed outdoor 2", "Fixed fluorescent 1", "Fixed fluorescent 2", "Hold current"]}, {["Auto", "Flicker-free 50 Hz", "Flicker-free 60 Hz", "Hold current"]}, {["None", "Prioritize frame rate", "Prioritize image quality"]}, {["Monochrome", "Color"]}] -> [_ _ _ _ _ w288]
          frame Default {
            w246 = FALSE ("Visible")
            w245 = FALSE ("Visible")
            n132 = property on="Motor" class="Clust (strict)"("Visible"=w245) -> ()  [unwired: 2 in, 2 out]
            n133 = property on="Test Ring" class="Ring (strict)"("Visible"=w245) -> ()  [unwired: 2 in, 2 out]
            n134 = property on="Rev/Fwd" class="Clust (strict)"("Visible"=w246) -> ()  [unwired: 2 in, 2 out]
            n135 = property on="On/Off" class="Bool (strict)"("Visible"=w246) -> ()  [unwired: 2 in, 2 out]
            n136 = property on="Test Slider" class="Slide (strict)"("Visible"=w246) -> ()  [unwired: 2 in, 2 out]
          }
          frame "Analog Out", "Motor", "PWM" {
            w252 = FALSE ("Visible")
            n137 = case shown="\"Analog Out\"" w251 {
              tunnel: [1.0 ("Value") -1.0 ("Value") 0.0 ("Value")] -> w250
              tunnel: [255.0 ("Value") 1.0 ("Value") 5.0 ("Value")] -> w249
              tunnel: [128.0 ("Value") 0.0 ("Value") 0.0 ("Value")] -> w248
              tunnel: [64.0 ("Value") 0.5 ("Value") 1.0 ("Value")] -> w247
              frame "PWM" {
              }
              frame "Motor", Default {
              }
              frame "Analog Out" {
              }
            }
            n138 = property on="Motor" class="Clust (strict)"("Visible"=TRUE) -> ()  [unwired: 2 in, 2 out]
            n139 = property on="Value" class="Slide (strict)"("Value"=w248, "Scale.Minimum"=w250, "Scale.Maximum"=w249, "Scale.Increment"=w247) -> ()  [unwired: 2 in, 2 out]
            n140 = property on="On/Off" class="Bool (strict)"("Visible"=w252) -> ()  [unwired: 2 in, 2 out]
            n141 = property on="Test Slider" class="Slide (strict)"("Visible"=w252) -> ()  [unwired: 2 in, 2 out]
            n142 = property on="Test Ring" class="Ring (strict)"("Visible"=w252) -> ()  [unwired: 2 in, 2 out]
            n143 = property on="Rev/Fwd" class="Clust (strict)"("Visible"=w252) -> ()  [unwired: 2 in, 2 out]
          }
          frame "Servo" {
            w268 = FALSE ("Visible")
            n144 = call <vilib>:"NT Read Number.vi"("Name"=w270) -> ("Numeric"=w269:dbl)  [unwired: 9 in, 1 out]
            n145 = property on="Test Slider" class="Slide (strict)"("Visible"=TRUE, "Scale.Maximum"=170.0 ("Scale.Range:Maximum")) -> ()  [unwired: 2 in, 2 out]
            n146 = local write "Test Slider"(w269) -> ()
            n147 = property on="Motor" class="Clust (strict)"("Visible"=w268) -> ()  [unwired: 2 in, 2 out]
            n148 = property on="Rev/Fwd" class="Clust (strict)"("Visible"=w268) -> ()  [unwired: 2 in, 2 out]
            n149 = property on="On/Off" class="Bool (strict)"("Visible"=w268) -> ()  [unwired: 2 in, 2 out]
            n150 = property on="Test Ring" class="Ring (strict)"("Visible"=w268) -> ()  [unwired: 2 in, 2 out]
          }
          frame "Relay", "Solenoid" {
            w271 = FALSE ("Visible")
            n151 = property on="Motor" class="Clust (strict)"("Visible"=w271) -> ()  [unwired: 2 in, 2 out]
            n152 = property on="Test Slider" class="Slide (strict)"("Visible"=w271) -> ()  [unwired: 2 in, 2 out]
            n153 = Search and Replace String(input string=w272, search string="/Value  **", replace string="/Direction") -> (result string=w278:string)  [unwired: 5 in, 3 out]
            n154 = property on="Test Ring" class="Ring (strict)"("Visible"=w271) -> ()  [unwired: 2 in, 2 out]
            n155 = call <vilib>:"NT Read String.vi"("Name"=w278) -> ("String"=w276:string)  [unwired: 9 in, 1 out]
            n156 = Equal?(x="Both directions", y=w276) -> (x = y?=w274:bool)
            n157 = Not(x=w274) -> (.not. x?=w275:bool)
            n158 = property on="Rev/Fwd" class="Clust (strict)"("Visible"=w274) -> ()  [unwired: 2 in, 2 out]
            n159 = property on="On/Off" class="Bool (strict)"("Visible"=w275, "Caption.Text"=w273) -> ()  [unwired: 2 in, 2 out]
          }
          frame "Compressor", "Digital Out" {
            w281 = FALSE ("Visible")
            # "Get direction and finish"
            n160 = property on="Motor" class="Clust (strict)"("Visible"=w281) -> ()  [unwired: 2 in, 2 out]
            n161 = property on="Test Slider" class="Slide (strict)"("Visible"=w281) -> ()  [unwired: 2 in, 2 out]
            n162 = property on="Test Ring" class="Ring (strict)"("Visible"=w281) -> ()  [unwired: 2 in, 2 out]
            n163 = property on="On/Off" class="Bool (strict)"("Visible"=TRUE, "Caption.Text"=w282) -> ()  [unwired: 2 in, 2 out]
            n164 = property on="Rev/Fwd" class="Clust (strict)"("Visible"=FALSE) -> ()  [unwired: 2 in, 2 out]
          }
          frame "Camera" {
            n165 = call <vilib>:"Get Last Path Segment.vi"("String in"=w289) -> ("String out"=w290:string)  [unwired: 10 in]
            n166 = property on="On/Off" class="Bool (strict)"("Visible"=FALSE) -> ()  [unwired: 2 in, 2 out]
            n167 = property on="Motor" class="Clust (strict)"("Visible"=FALSE) -> ()  [unwired: 2 in, 2 out]
            n168 = property on="Rev/Fwd" class="Clust (strict)"("Visible"=FALSE) -> ()  [unwired: 2 in, 2 out]
            n169 = case shown="\"White Balance  **\"" w290 {
              tunnel: w289 -> [w296 w305 w314 w323 w332 _ w338]
              tunnel: w288 -> [w294 w302 w311 w320 w329 _ _]
              frame "Size  **" {
                n170 = Index Array(array=w294) -> (element=w293:cluster{string[]})  [unwired: 1 in]
                n171 = call <vilib>:"NT Read String.vi"("Name"=w296) -> ("String"=w295:string)  [unwired: 9 in, 1 out]
                n172 = Unbundle(w293) -> (w291:string[])
                n173 = Match First String(2:w291, 3:w295) -> (0:w292:i32)  [unwired: 1 out]
                n174 = property on="Test Ring" class="Ring (strict)"("Value"=w292, "Strings []"=w291) -> ()  [unwired: 2 in, 2 out]
                n175 = property on="Test Ring" class="Ring (strict)"("Visible"=TRUE) -> ()  [unwired: 2 in, 2 out]
                n176 = property on="Test Slider" class="Slide (strict)"("Visible"=FALSE) -> ()  [unwired: 2 in, 2 out]
              }
              frame "White Balance  **" {
                n177 = Index Array(array=w302, index=1) -> (element=w303:cluster{string[]})
                n178 = call <vilib>:"NT Read String.vi"("Name"=w305) -> ("String"=w304:string)  [unwired: 9 in, 1 out]
                n179 = Unbundle(w303) -> (w300:string[])
                n180 = Match First String(2:w300, 3:w304) -> (0:w299:i32)  [unwired: 1 out]
                n181 = property on="Test Ring" class="Ring (strict)"("Value"=w299, "Strings []"=w300) -> ()  [unwired: 2 in, 2 out]
                n182 = property on="Test Ring" class="Ring (strict)"("Visible"=TRUE) -> ()  [unwired: 2 in, 2 out]
                n183 = property on="Test Slider" class="Slide (strict)"("Visible"=FALSE) -> ()  [unwired: 2 in, 2 out]
              }
              frame "Exposure  **" {
                n184 = Index Array(array=w311, index=2) -> (element=w312:cluster{string[]})
                n185 = call <vilib>:"NT Read String.vi"("Name"=w314) -> ("String"=w313:string)  [unwired: 9 in, 1 out]
                n186 = Unbundle(w312) -> (w308:string[])
                n187 = Match First String(2:w308, 3:w313) -> (0:w309:i32)  [unwired: 1 out]
                n188 = property on="Test Ring" class="Ring (strict)"("Value"=w309, "Strings []"=w308) -> ()  [unwired: 2 in, 2 out]
                n189 = property on="Test Ring" class="Ring (strict)"("Visible"=TRUE) -> ()  [unwired: 2 in, 2 out]
                n190 = property on="Test Slider" class="Slide (strict)"("Visible"=FALSE) -> ()  [unwired: 2 in, 2 out]
              }
              frame "Exposure Priority  **" {
                n191 = Index Array(array=w320, index=3) -> (element=w321:cluster{string[]})
                n192 = call <vilib>:"NT Read String.vi"("Name"=w323) -> ("String"=w322:string)  [unwired: 9 in, 1 out]
                n193 = Unbundle(w321) -> (w317:string[])
                n194 = Match First String(2:w317, 3:w322) -> (0:w318:i32)  [unwired: 1 out]
                n195 = property on="Test Ring" class="Ring (strict)"("Value"=w318, "Strings []"=w317) -> ()  [unwired: 2 in, 2 out]
                n196 = property on="Test Ring" class="Ring (strict)"("Visible"=TRUE) -> ()  [unwired: 2 in, 2 out]
                n197 = property on="Test Slider" class="Slide (strict)"("Visible"=FALSE) -> ()  [unwired: 2 in, 2 out]
              }
              frame "Color Enable  **" {
                n198 = Index Array(array=w329, index=4) -> (element=w330:cluster{string[]})
                n199 = call <vilib>:"NT Read String.vi"("Name"=w332) -> ("String"=w331:string)  [unwired: 9 in, 1 out]
                n200 = Unbundle(w330) -> (w326:string[])
                n201 = Match First String(2:w326, 3:w331) -> (0:w327:i32)  [unwired: 1 out]
                n202 = property on="Test Ring" class="Ring (strict)"("Value"=w327, "Strings []"=w326) -> ()  [unwired: 2 in, 2 out]
                n203 = property on="Test Ring" class="Ring (strict)"("Visible"=TRUE) -> ()  [unwired: 2 in, 2 out]
                n204 = property on="Test Slider" class="Slide (strict)"("Visible"=FALSE) -> ()  [unwired: 2 in, 2 out]
              }
              frame Default {
                n205 = property on="Test Ring" class="Ring (strict)"("Visible"=FALSE) -> ()  [unwired: 2 in, 2 out]
                n206 = property on="Test Slider" class="Slide (strict)"("Visible"=FALSE) -> ()  [unwired: 2 in, 2 out]
              }
              frame "Brightness  **", "Color Level  **", "Compression  **", "FPS  **", "Sharpness  **" {
                n207 = call <vilib>:"NT Read Number.vi"("Name"=w338) -> ("Numeric"=w337:dbl)  [unwired: 9 in, 1 out]
                n208 = local write "Test Slider"(w337) -> ()
                n209 = property on="Test Slider" class="Slide (strict)"("Visible"=TRUE, "Scale.Maximum"=100.0 ("Scale.Range:Maximum")) -> ()  [unwired: 2 in, 2 out]
                n210 = property on="Test Ring" class="Ring (strict)"("Visible"=FALSE) -> ()  [unwired: 2 in, 2 out]
              }
            }
          }
        }
        n211 = property on="Progress" class="Clust (strict)"("Visible"=FALSE) -> ()  [unwired: 2 in, 2 out]
      }
      event "Test Name": Mouse Enter {
        # "Populate the ring with the list of tests"
        n212 = event-data() -> ()  [unwired: 1 in, 1 out]
        n213 = call <vilib>:"NT Read String Array.vi"("Name"="TestMode/TestList") -> ("String Array"=w346:string[])  [unwired: 9 in, 1 out]
        n214 = Build Array (concatenate)("Select the test to run...", w346) -> (w345:string[])
        n215 = property on="Test Name" class="Ring (strict)"("Strings []"=w345) -> ()  [unwired: 2 in, 2 out]
      }
      event "Test Name": Value Change {
        w348 = FALSE ("Visible")
        # "Tell the robot the test name to run"
        n216 = event-data() -> ("NewVal"=w352:u16)  [unwired: 1 in]
        n217 = property on="Test Name" class="Ring (strict)"() -> ("Strings []"=w353:string[])  [unwired: 2 in, 2 out]
        n218 = local write "Progress"(T6 {"Test Progress"=0, "Test Progress Text"=""} ("Progress")) -> ()
        n219 = Index Array(array=w353, index=w352) -> (element=w351:string)
        n220 = call <vilib>:"NT Write String.vi"("String"=w351, "Name"="TestMode/TestName") -> ()  [unwired: 9 in, 1 out]
        n221 = property on="Progress" class="Clust (strict)"("Visible"=TRUE) -> ()  [unwired: 2 in, 2 out]
        n222 = property on="Motor" class="Clust (strict)"("Visible"=w348) -> ()  [unwired: 2 in, 2 out]
        n223 = property on="Test Slider" class="Slide (strict)"("Visible"=w348) -> ()  [unwired: 2 in, 2 out]
        n224 = property on="On/Off" class="Bool (strict)"("Visible"=w348) -> ()  [unwired: 2 in, 2 out]
        n225 = property on="Rev/Fwd" class="Clust (strict)"("Visible"=w348) -> ()  [unwired: 2 in, 2 out]
        n226 = property on="Test Ring" class="Ring (strict)"("Visible"=w348) -> ()  [unwired: 2 in, 2 out]
      }
      event "Select Auto": Mouse Enter {
        # "Populate the combo box with the list of autonomous options"
        n227 = event-data() -> ()  [unwired: 1 in, 1 out]
        n228 = call <vilib>:"NT Read String Array.vi"("Name"="Auto List") -> ("String Array"=w355:string[])  [unwired: 9 in, 1 out]
        n229 = property on="Select Auto" class="CmbBox"("Strings[]"=w355) -> ()  [unwired: 2 in, 2 out]
      }
      event "Select Auto": Value Change {
        # "User modified the Auto Selection. Write to NT variable so robot knows."
        n230 = event-data() -> ("NewVal"=w358:string)  [unwired: 1 in]
        n231 = call <vilib>:"NT Write String.vi"("String"=w358, "Name"="Auto Selector") -> ()  [unwired: 9 in, 1 out]
      }
      event "Command Selection": Value Change {
        # "Get the params and show in table"
        n232 = event-data() -> ("NewVal"=w364:i32)  [unwired: 1 in]
        n233 = property on="Command Selection" class="MCListbox (strict)"() -> ("ItemNames"=w362:string[][])  [unwired: 2 in, 2 out]
        n234 = call <vilib>:"WPI_DashboardUpdate Command Params.vi"("NewVal"=w364, "Commands"=w362, "Param Tbl"=w363) -> ()  [unwired: 8 in, 1 out]
      }
      event "Execute Command": Value Change {
        # "Started one, Unique ID holds\nresponse"
        n235 = event-data() -> ()  [unwired: 1 in, 1 out]
        n236 = property on="Command Selection" class="MCListbox (strict)"() -> ("ItemNames"=w375:string[][])  [unwired: 2 in, 2 out]
        n237 = Index Array(array=w375, index (row)="Command Selection", index (col)=0) -> (element=w373:string)
        n238 = call <vilib>:"Invoke Commands.vi"("Command Params"="Command Params", "Function Name"=w373) -> ("Params"=w369:u8, "Started"=w368:bool)  [unwired: 7 in, 1 out]
        n239 = Array Subset(array="Command Params", length (row)=w369) -> (w370:string[][])  [unwired: 3 in]
        n240 = Select(t="Executing" ("Cmd Status"), s=w368, f="" ("Cmd Status")) -> (s? t:f=→"Cmd Status":string)
      }
      event "Command Selection": Double Click {
        n241 = event-data() -> ("Row"=w383:i32)  [unwired: 1 in]
        n242 = property on="Command Selection" class="MCListbox (strict)"() -> ("ItemNames"=w386:string[][])  [unwired: 2 in, 2 out]
        n243 = local read "Command Params"() -> (w382:string[][])
        n244 = Index Array(array=w386, index (row)=w383, index (col)=0) -> (element=w384:string)
        n245 = call <vilib>:"Invoke Commands.vi"("Command Params"=w382, "Function Name"=w384) -> ("Params"=w381:u8, "Started"=w376:bool)  [unwired: 7 in, 1 out]
        n246 = Array Subset(array=w382, length (row)=w381) -> (w380:string[][])  [unwired: 3 in]
        n247 = Select(t="Executing" ("Cmd Status"), s=w376, f="" ("Cmd Status")) -> (s? t:f=w377:string)
        n248 = local write "Cmd Status"(w377) -> ()
      }
      event "CheckList": Double Click {
        # "Shift clears all"
        # "Update symbols on the listbox"
        n249 = event-data() -> ("PlatMods.Shift"=w388:bool, "Row"=w390:i32)  [unwired: 1 in]
        n250 = case shown="True" w388 {
          tunnel: w390 -> [w394 _]
          tunnel: 1 -> [w393 _]
          frame False {
            n251 = property on="CheckList" class="LstBox (strict)"() -> ("Item Symbols"=w392:i32[])  [unwired: 2 in, 2 out]
            n252 = Replace Array Subset(array=w392, new element=w393, index=w394) -> (w391:i32[])
            n253 = property on="CheckList" class="LstBox (strict)"("Item Symbols"=w391) -> ()  [unwired: 2 in, 2 out]
          }
          frame True {
            w395 = 0 ("Top Row")
            n254 = property on="CheckList" class="LstBox (strict)"() -> ("Number of Rows"=w397:u32)  [unwired: 2 in, 2 out]
            n255 = Initialize Array(0, w397) -> (w396:i32[])
            n256 = property on="CheckList" class="LstBox (strict)"("Top Row"=w395, "Value"=w395, "Item Symbols"=w396) -> ()  [unwired: 2 in, 2 out]
          }
        }
      }
      event "CheckList": Key Down {
        # "Update symbols on the listbox\nLeft and right keys check and uncheck"
        n257 = event-data() -> ("VKey"=w401:T23)  [unwired: 1 in]
        n258 = case shown="\"Left\", \"Right\"" w401 {
          selector: w401 -> [w406 _]
          tunnel: eventvkey."Left" ("VKey") -> [w404 _]
          frame "Left", "Right" {
            n259 = Equal?(x=w404, y=w406) -> (x = y?=w405:bool)
            n260 = Select(t=0, s=w405, f=1) -> (s? t:f=w407:i32)
            n261 = property on="CheckList" class="LstBox (strict)"() -> ("Item Symbols"=w410:i32[])  [unwired: 2 in, 2 out]
            n262 = Replace Array Subset(array=w410, new element=w407, index="CheckList") -> (w409:i32[])
            n263 = property on="CheckList" class="LstBox (strict)"("Item Symbols"=w409) -> ()  [unwired: 2 in, 2 out]
          }
          frame Default {
          }
        }
      }
      event "Motor.Enable": Value Change {
        # "When the test mode otor enable helper is set, update that\ntree row item's value"
        n264 = event-data() -> ("NewVal"=w416:bool)  [unwired: 1 in]
        n265 = Unbundle("Motor") -> ("Value"=w415:dbl)  [unwired: 1 out]
        n266 = Select(t=w415, s=w416, f=0.0) -> (s? t:f=w413:dbl)
        n267 = call <vilib>:"NT Write Number.vi"("Numeric"=w413, "Name"=w412) -> ()  [unwired: 9 in, 1 out]
      }
      event "Test Slider": Value Change {
        # "When the test mode slider helper is set, update that\ntree row item's value"
        n268 = event-data() -> ("NewVal"=w419:dbl)  [unwired: 1 in]
        n269 = call <vilib>:"NT Write Number.vi"("Numeric"=w419, "Name"=w420) -> ()  [unwired: 9 in, 1 out]
      }
      event "On/Off": Value Change {
        # "When the test mode on/off helper value is set, update that\ntree row item's value"
        n270 = event-data() -> ("NewVal"=w424:bool)  [unwired: 1 in]
        n271 = Boolean To (0,1)(Boolean=w424) -> (0, 1=w423:i16)
        n272 = call <vilib>:"NT Write Number.vi"("Numeric"=w423, "Name"=w422) -> ()  [unwired: 9 in, 1 out]
      }
      event "Rev/Fwd": Value Change {
        # "When the test mode helper value for relays is set, update that\ntree row item's value"
        n273 = event-data() -> ("NewVal.Forward"=w432:bool, "NewVal.Reverse"=w431:bool)  [unwired: 1 in]
        n274 = Boolean To (0,1)(Boolean=w432) -> (0, 1=w428:i16)
        n275 = Boolean To (0,1)(Boolean=w431) -> (0, 1=w430:i16)
        n276 = Negate(x=w430) -> (-x=w429:i16)
        n277 = Add(x=w428, y=w429) -> (x+y=w427:i16)
        n278 = call <vilib>:"NT Write Number.vi"("Numeric"=w427, "Name"=w426) -> ()  [unwired: 9 in, 1 out]
      }
      event "Test Ring": Value Change {
        # "When a test mode helper value is selected from the ring,\nset the tree item's variable to the string value"
        n279 = event-data() -> ("NewVal"=w436:u16)  [unwired: 1 in]
        n280 = property on="Test Ring" class="Ring (strict)"() -> ("Strings []"=w437:string[])  [unwired: 2 in, 2 out]
        n281 = Index Array(array=w437, index=w436) -> (element=w435:string)
        n282 = call <vilib>:"NT Write String.vi"("String"=w435, "Name"=w434) -> ()  [unwired: 9 in, 1 out]
      }
      event "Rec Mode": Value Change {
        # "Update globals for recording mode and path to read log from.\nClear when logging and let NetworkTables set path for vision to\nuse."
        n283 = event-data() -> ("NewVal"=w448:enum32{"Stop", "Record", "Playback"})  [unwired: 1 in]
        n284 = global write "WPI_DashboardLogging Global.vi" "Logging Filename"(path "") -> ()
        n285 = global write "WPI_DashboardLogging Global.vi" "Recording"(w448) -> ()
        n286 = case shown="\"Playback\"" w448 {
          tunnel: w447 -> [_ w450 w459]
          tunnel: [_ _ w458] -> w445
          tunnel: [_ _ w457] -> _
          tunnel: w443 -> [_ _ w455]
          tunnel: cluster{i32, i32} {-250, 170} -> [_ _ w454]
          tunnel: [_ _ T24 {"Image Size"=TRUE, "Image Type"=TRUE, "Pixel Value"=TRUE, "ROI Information"=TRUE, "Zoom Factor"=FALSE} ("Image Information Shown:All Elements")] -> w438
          tunnel: [_ _ TRUE ("Zoom Factor")] -> w439
          tunnel: w441 -> [_ _ w451]
          frame Default {
          }
          frame "Stop", "Record" {
            # "Place Window too"
            n287 = invoke class="VI" method="FP.Close"(reference=w450) -> (reference out=w449:refnum<vi>)  [unwired: 2 in, 2 out]
            n288 = invoke class="VI" method="Abort VI"(reference=w449) -> ()  [unwired: 2 in, 3 out]
          }
          frame "Playback" {
            n289 = call "Open Playback Panel.vi"("Offset"=w454, "DB VI Ref"=w455, "Playback in"=w459) -> ("Playback out"=w456:refnum<vi>)  [unwired: 8 in]
            n290 = register-events(w456, w451) -> (reference out=w458:refnum<event-registration>, error out=w457:errorcluster)  [unwired: 2 in]
          }
        }
        n291 = property on="Camera Image Right" class="ImageControl"("Image Information Shown"=w438, "Image Information Visible"=w439) -> ()  [unwired: 2 in, 2 out]
        n292 = property on="Camera Image" class="ImageControl"("Image Information Shown"=w438, "Image Information Visible"=w439) -> ()  [unwired: 2 in, 2 out]
        n293 = call <vilib>:"WPI_DashboardNT Log FieldName Cache.vi"("Operation"=enum16{"Lookup/Add", "Index", "Clear"}."Clear") -> ()  [unwired: 8 in, 3 out]
      }
      event Panel Close {
        w461 = enum32{"Stop", "Record", "Playback"}."Stop" ("Rec Mode")
        # "Playback window has been closed, abort"
        n294 = event-data() -> ()  [unwired: 1 in, 4 out]
        n295 = local write "Rec Mode"(w461) -> ()
        n296 = global write "WPI_DashboardLogging Global.vi" "Recording"(w461) -> ()
      }
      event Panel Close {
        # "Abort playback window and ourself"
        n297 = event-data() -> ()  [unwired: 1 in, 4 out]
        n298 = invoke class="VI" method="FP.Close"(reference=w465) -> (reference out=w464:refnum<vi>)  [unwired: 2 in, 2 out]
        n299 = invoke class="VI" method="Abort VI"(reference=w464) -> (error out=w463:errorcluster)  [unwired: 2 in, 2 out]
        n300 = invoke class="VI" method="Abort VI"(error in=w463) -> ()  [unwired: 2 in, 3 out]
      }
      event User Event {
        n301 = event-data() -> ("IDs"=w472:cluster{"RPC field ID":u16, "Unique ID":u16}, "String"=w471:string)  [unwired: 1 in]
        n302 = Bundle("IDs"=w472, "String"=w471) -> (w470:T10)  [unwired: 1 in]
        n303 = call <vilib>:"Retrieve RPC Response.vi"("RPC Response"=w470) -> ("Output"=w468:string[][])  [unwired: 10 in]
        n304 = Build Array (concatenate)(w466, w468) -> (w467:string[][])
        n305 = local write "Command Params"(w467) -> ()
        n306 = local write "Cmd Status"("" ("Cmd Status")) -> ()
      }
      event "Tree": Double Click {
        n307 = event-data() -> ("PlatMods"=w478:T27, "Tag"=w475:string)  [unwired: 1 in]
        n308 = Unbundle(w478) -> ("Shift"=w477:bool)  [unwired: 4 out]
        n309 = String Subset(string=w475, length (rest)=1 ("length (rest)")) -> (substring=w474:string)  [unwired: 1 in]
        n310 = Not(x=w477) -> (.not. x?=w476:bool)
        n311 = case shown="\"/\"" w474 {
          tunnel: w475 -> [_ w481]
          tunnel: w476 -> [_ w480]
          frame Default {
          }
          frame "/" {
            n312 = call <vilib>:"NT Update Persistence.vi"("Persistence"=w480, "Name"=w481) -> ()  [unwired: 9 in, 1 out]
          }
        }
      }
    }
  }
  n313 = while {
    tunnel: w67 -> [w483]
    i -> [w486]
    stop <- FALSE stop-if-true
    n314 = Wait (ms)(milliseconds to wait=u32 100) -> ()  [unwired: 1 out]
    n315 = case shown="\"Playback\"" "Rec Mode" {
      tunnel: w486 -> [_ _ w501]
      tunnel: [u32 2829099 ("Base Color") u32 11141120 ("Target Color") w490] -> w482
      frame "Stop", Default {
        # "Reset the color, extra updates don't cost much"
      }
      frame "Record" {
      }
      frame "Playback" {
        # "Playback"
        n316 = Quotient & Remainder(x=w501, y=u32 50 ("milliseconds to wait")) -> (x-y*floor(x/y)=w497:u32)  [unwired: 1 out]
        n317 = Divide(x=w497, y=u32 50 ("milliseconds to wait")) -> (x/y=w494:dbl)
        n318 = Multiply(x=6.283185307179586, y=w494) -> (x*y=w499:dbl)
        n319 = Sine(x=w499) -> (sin(x)=w498:dbl)
        n320 = Absolute Value(x=w498) -> (abs(x)=w491:dbl)
        n321 = call "Interpolate RGB Color.vi"("Proportion"=w491, "Target Color"=u32 30976, "Base Color"=u32 2829099) -> ("Result Color"=w490:u32)  [unwired: 8 in]
      }
    }
    n322 = property class="Pane"(reference=w483, "PaneColor"=w482) -> ()  [unwired: 1 in, 2 out]
  }
  n323 = local write "Dashboard Tab"(T2."Drive" ("Dashboard Tab")) -> ()
  n324 = property on="On/Off" class="Bool (strict)"("Visible"=w40) -> ()  [unwired: 2 in, 2 out]
  n325 = property on="Motor" class="Clust (strict)"("Visible"=w40) -> ()  [unwired: 2 in, 2 out]
  n326 = property on="Progress" class="Clust (strict)"("Visible"=w40) -> ()  [unwired: 2 in, 2 out]
  n327 = property on="Test Ring" class="Ring (strict)"("Visible"=w40) -> ()  [unwired: 2 in, 2 out]
  n328 = property on="Rev/Fwd" class="Clust (strict)"("Visible"=w40) -> ()  [unwired: 2 in, 2 out]
  n329 = while {
    tunnel: u16 1741 ("timeout ms (25000)") -> [w503]
    stop <- FALSE stop-if-true
    n330 = TCP Create Listener(10:w503) -> (0:w502:errorcluster, 3:w504:refnum<k5>)  [unwired: 4 in, 1 out]
    n331 = case shown="No Error" w502 {
      selector: w502 -> [w506 _]
      tunnel: w504 -> [w507 _]
      frame No Error {
        n332 = while {
          tunnel: w507 -> [w510]
          tunnel: w506 -> [w509]
          stop <- FALSE stop-if-true
          n333 = TCP Wait On Listener(8:w509, 11:w510) -> (0:w511:errorcluster, 4:w512:refnum<k5>)  [unwired: 2 in, 3 out]
          n334 = local write "TCP"(w512) -> ()
          n335 = case shown="No Error" w511 {
            frame No Error {
            }
            frame Error {
              n336 = Wait (ms)(milliseconds to wait=u32 1000) -> ()  [unwired: 1 out]
            }
          }
        }
      }
      frame Error {
        n337 = Wait (ms)(milliseconds to wait=u32 1000) -> ()  [unwired: 1 out]
      }
    }
  }
  n338 = local write "Command Selection"(u16 0 ("milliseconds to wait")) -> ()
  n339 = local write "Command Params"(string[][] [] ("Command Params")) -> ()
  n340 = global write "WPI_DashboardLogging Global.vi" "Recording"(w61) -> ()
  n341 = local write "Rec Mode"(w61) -> ()
  n342 = call <vilib>:"NT Write String.vi"("String"="Select Auto", "Name"="Auto Selector") -> ()  [unwired: 9 in, 1 out]
